vi "Acquisition_BassShaker.vi"() -> ()   [LabVIEW 2017]
uses:
  <vilib>/Utility/error.llb/DialogType.ctl
  <vilib>/DAQmx/write.llb/DAQmx Write (Digital Bool 1Line 1Point).vi
  <vilib>/DAQmx/read.llb/DAQmx Read (Analog 1D Wfm NChan NSamp).vi
  <vilib>/Utility/file.llb/Write Delimited Spreadsheet (DBL).vi
panel:
  in  "Activity Based On:":u16(ring) items=["EMG", "Piezo"]
  in  "Piezo Filter Parameters File:":path=path "C:/Users/local_admin/Desktop/Sleep Modulation/Piezo_Coefs.csv"
  in  "AO Channel":tag="Dev3/ao0"
  out "Stim":bool
  in  "Stim?":bool
  out "Detection":bool
  in  "Stop":bool
  in  "Target State:":u16(ring)=3 items=["Wake"=1, "NREM"=2, "REM"=3]
  in  "Frequency":dbl=50.0 format="%0.2p"
  in  "Amplitude":dbl=0.2 format="%0.2p"
  in  "Preamp Gain:":u16(ring)=10 items=["10X"=10, "100X"=100]
  in  "Modeling":u16(ring)=1 items=["Building", "Implementing"]
  out "Predicted State":i32(ring)=1 items=["Wake"=1, "NREM"=2, "REM"=3]
  in  "Minimum\nDuration":dbl=5.0
  in  "Feature Save To Path":path=path "C:/Users/local_admin/Desktop/Shaker Trials/NSL39/50Hz, 200mV/NSL39_50Hz200mV.csv"
  in  "EEG Filter Parameters File:":path=path "C:/Users/local_admin/Desktop/Sleep Modulation/EEG_Coefs.csv"
  in  "Model Information File (Mu, Sigma, Priors, Transition Matrix):":path=path "C:/Users/local_admin/Desktop/Shaker Trials/NSL39/Model_NSL39_10072017.csv"
  out "EEG":waveform(dbl)(graph)={"t0"=timestamp(3591178838.0438023 s since 1904-01-01), "dt"=0.0025, "Y"=array[400 elements], "attributes"=variant("NI_ChannelName"=variant(string "EEG"), "NI_UnitDescription"=variant(string "Volts"))}
  out "Piezo":waveform(dbl)(graph)={"t0"=timestamp(0 s since 1904-01-01), "dt"=1.0, "Y"=array[400 elements]}
  # "STIMULATION SETTINGS"
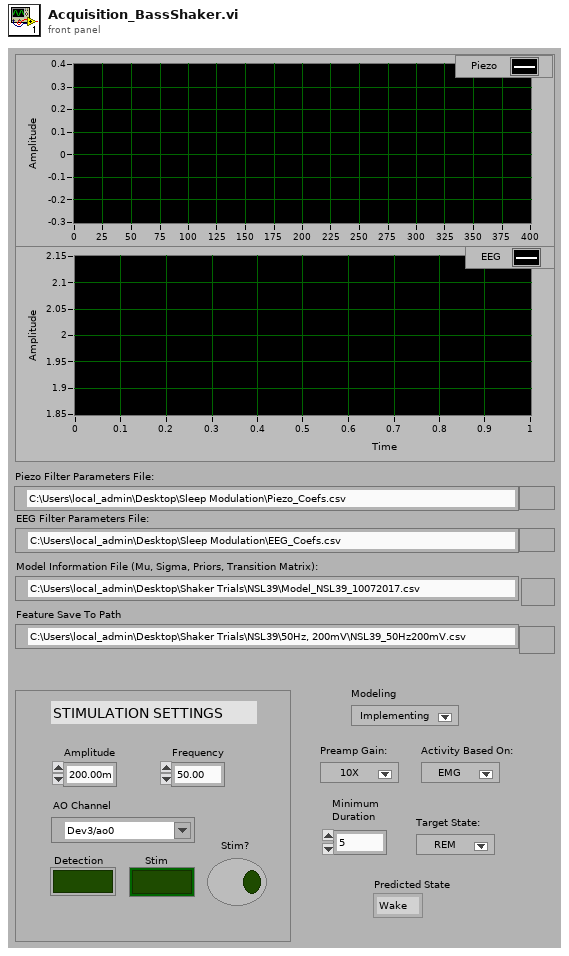
[diagram p1: front panel]
types:
  T1 = typedef "DialogType.ctl" = u16
  T2 = typedef "TYPE EEG Components.ctl" = cluster{"Total":dbl, "Alpha":dbl, "Beta":dbl, "Gamma":dbl, "Delta":dbl, "Delta Low":dbl, "Delta High":dbl, "Theta":dbl}
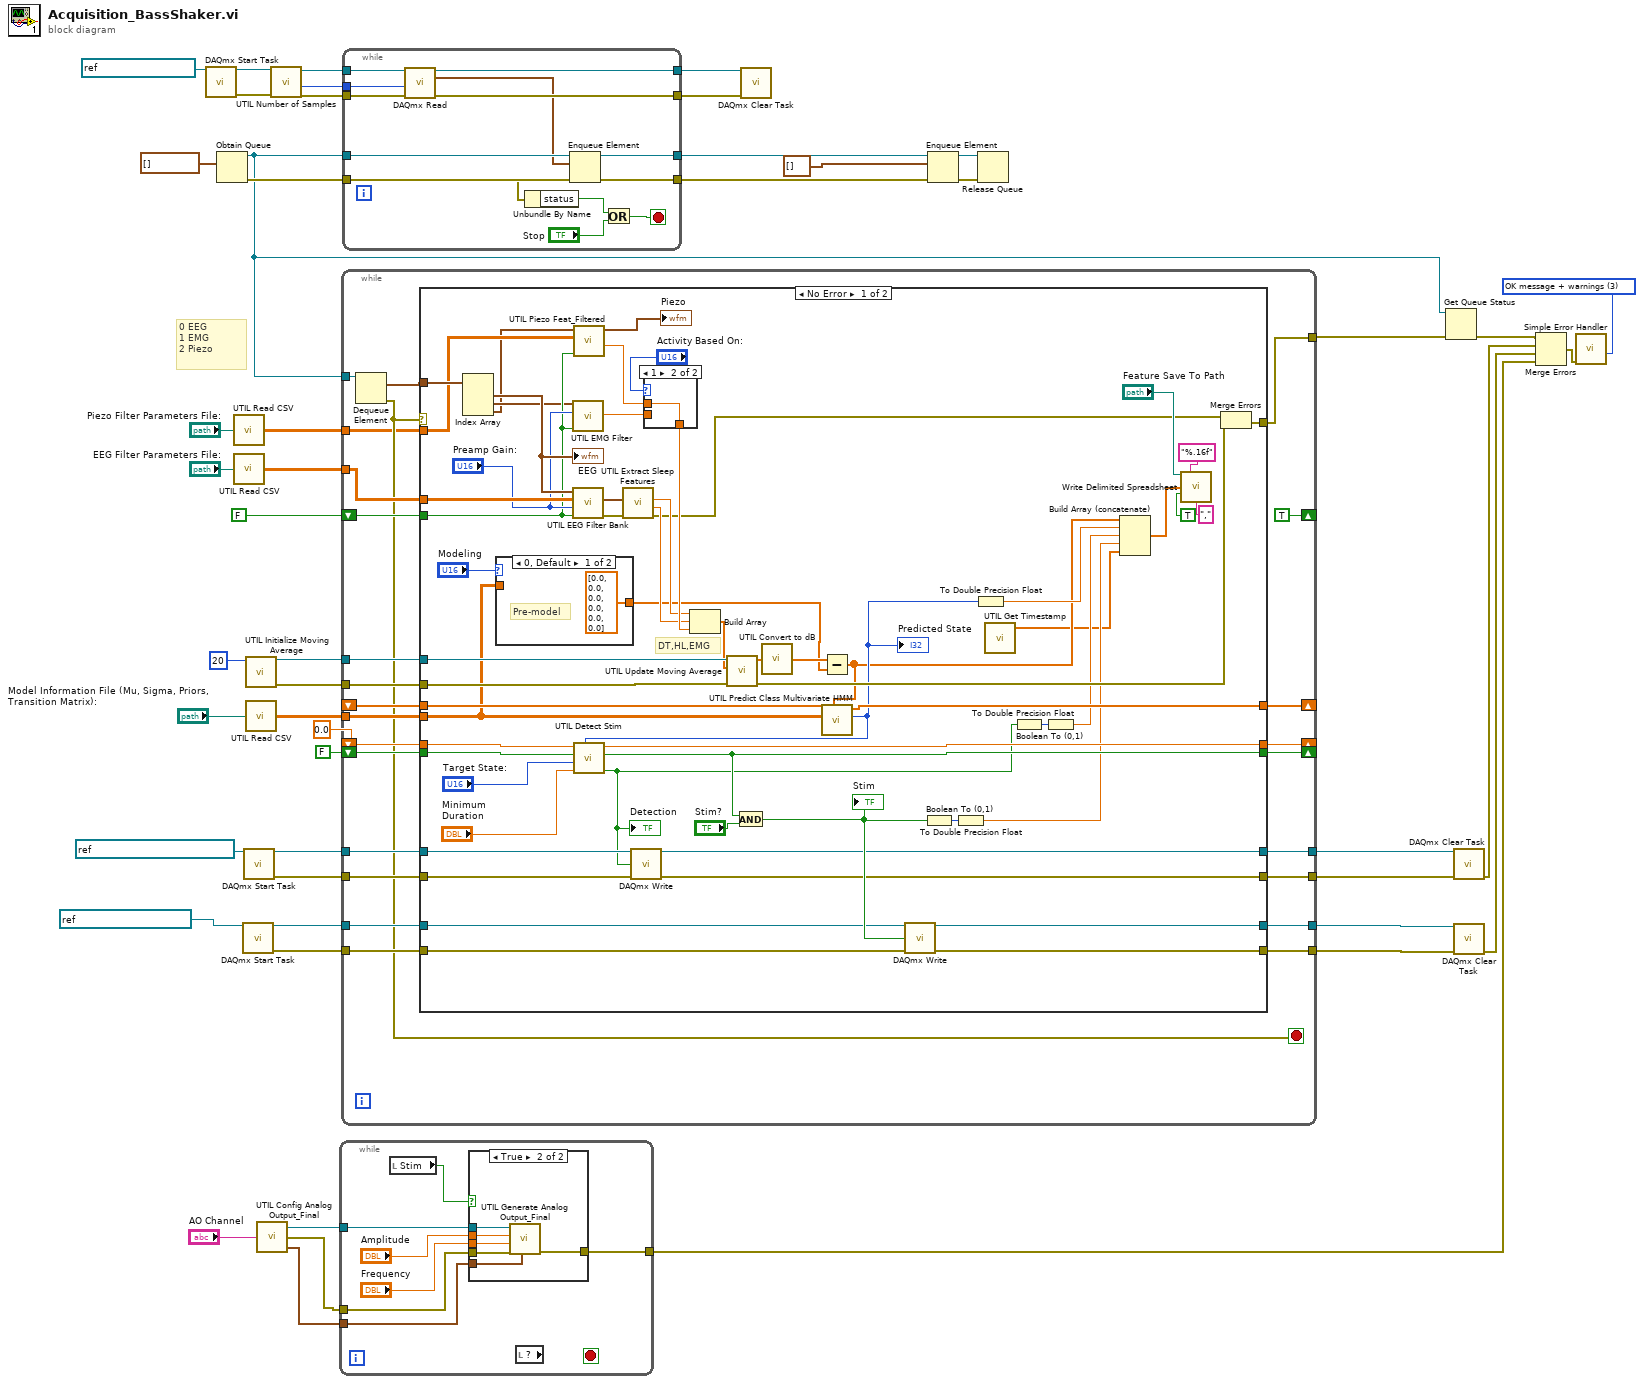
[diagram p0: block diagram]
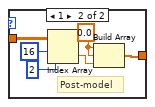
[diagram p3: hidden frame]
diagram:
  w42 = T1 3 items=["no dialog", "OK message", "continue or stop message", "OK message + warnings", "continue/stop + warnings"] ("type of dialog (OK msg:1)")
  # "0 EEG\n1 EMG\n2 Piezo"
  n1 = call <vilib>:"DAQmx Start Task.vi"("task/channels in"=refnum<k21> "BassShakerInput") -> ("task out"=w37:refnum<k21>, "error out"=w36:errorcluster)  [unwired: 13 in]
  n2 = Obtain Queue(element data type=waveform(dbl)[] [] ("Measurement 2")) -> (queue out=w3:refnum<queue>, error out=w48:errorcluster)  [unwired: 4 in, 1 out]
  n3 = call "UTIL Read CSV.vi"("CSV Path"="Piezo Filter Parameters File:") -> ("Data From File"=w1:dbl[][])
  n4 = call "UTIL Read CSV.vi"("CSV Path"="EEG Filter Parameters File:") -> ("Data From File"=w26:dbl[][])
  n5 = call <vilib>:"DAQmx Start Task.vi"("task/channels in"=refnum<k21> "StimAnnotationOut") -> ("task out"=w20:refnum<k21>, "error out"=w19:errorcluster)  [unwired: 13 in]
  n6 = call <vilib>:"DAQmx Start Task.vi"("task/channels in"=refnum<k21> "DetectionAnnotationOut") -> ("task out"=w23:refnum<k21>, "error out"=w22:errorcluster)  [unwired: 13 in]
  n7 = call "UTIL Initialize Moving Average.vi"("Window Width"=20) -> ("Error Out"=w29:errorcluster, "queue out"=w27:refnum<queue>)  [unwired: 9 in]
  n8 = call "UTIL Read CSV.vi"("CSV Path"="Model Information File (Mu, Sigma, Priors, Transition Matrix):") -> ("Data From File"=w39:dbl[][])
  n9 = call "UTIL Config Analog Output_Final.vi"("physical channels"="AO Channel") -> ("sampling info"=w10:cluster{"Fs":dbl, "#s":dbl}, "error out"=w8:errorcluster, "task out"=w7:refnum<k21>)
  n10 = call "UTIL Number of Samples.vi"("Error In"=w36, "Task In"=w37) -> ("Error Out"=w32:errorcluster, "Samples/Chan"=w33:i32, "Task Out"=w34:refnum<k21>)  [unwired: 7 in]
  n11 = while {
    tunnel: w10 -> [w54]
    tunnel: w8 -> [w53]
    tunnel: w7 -> [w52]
    tunnel: [w51] -> w6
    stop <- _ stop-if-true
    n12 = local read "Stim"() -> (w50:bool)
    n13 = case shown="True" w50 {
      tunnel: "Amplitude" -> [_ w63]
      tunnel: "Frequency" -> [_ w62]
      tunnel: w54 -> [_ w61]
      tunnel: w53 -> [w57 w60]
      tunnel: w52 -> [_ w59]
      tunnel: [w57 w58] -> w51
      frame False {
      }
      frame True {
        n14 = call "UTIL Generate Analog Output_Final.vi"("sampling info"=w61, "error in (no error)"=w60, "frequency"=w62, "amplitude"=w63, "task/channels in"=w59) -> ("error out"=w58:errorcluster)  [unwired: 5 in, 1 out]
      }
    }
    n15 = local read item#-1() -> ()  [unwired: 1 out]
  }
  n16 = while {
    tunnel: w3 -> [w87]
    shift-right: [TRUE] -> _
    shift-left: FALSE -> [w85]
    tunnel: [w81] -> w4
    tunnel: w29 -> [w84]
    tunnel: w39 -> [w83]
    tunnel: w26 -> [w82]
    tunnel: w27 -> [w80]
    shift-right: [w79] -> _
    shift-left: _ -> [w78]
    shift-right: [w76] -> _
    shift-left: 0.0 ("Detection Duration Out") -> [w77]
    shift-right: [w74] -> _
    shift-left: FALSE ("Stim State Out") -> [w75]
    tunnel: w23 -> [w73]
    tunnel: w22 -> [w72]
    tunnel: w20 -> [w71]
    tunnel: w19 -> [w70]
    tunnel: [w69] -> w18
    tunnel: [w68] -> w17
    tunnel: [w67] -> w16
    tunnel: [w66] -> w15
    tunnel: w1 -> [w64]
    stop <- w65 stop-if-true
    n17 = Dequeue Element(queue=w87) -> (element=w88:waveform(dbl)[], error out=w65:errorcluster)  [unwired: 2 in, 2 out]
    n18 = case shown="No Error" w65 {
      selector: w65 -> [_ w158]
      tunnel: w88 -> [w128 _]
      tunnel: w85 -> [w94 _]
      tunnel: [w142 w158] -> w81
      tunnel: w84 -> [w139 _]
      tunnel: w83 -> [w127 _]
      tunnel: w82 -> [w141 _]
      tunnel: w80 -> [w137 _]
      tunnel: [w136 w165] -> w79
      tunnel: w78 -> [w135 w165]
      tunnel: w77 -> [w123 w160]
      tunnel: [w122 w160] -> w76
      tunnel: w75 -> [w121 w159]
      tunnel: [w108 w159] -> w74
      tunnel: w73 -> [w119 w162]
      tunnel: w72 -> [w118 w161]
      tunnel: w71 -> [w114 w164]
      tunnel: w70 -> [w113 w163]
      tunnel: [w112 w164] -> w69
      tunnel: [w111 w163] -> w68
      tunnel: [w110 w162] -> w67
      tunnel: [w109 w161] -> w66
      tunnel: w64 -> [w95 _]
      frame No Error {
        # "DT,HL,EMG"
        n19 = Index Array(array=w128) -> (element #1=w106:waveform(dbl), element #2=w91:waveform(dbl), element #3=w90:waveform(dbl))  [unwired: 3 in]
        "EEG" <- w106
        n20 = case shown="0, Default" "Modeling" {
          tunnel: w127 -> [_ w155]
          tunnel: [dbl[] [0.0, 0.0, 0.0, 0.0, 0.0, 0.0] ("Parameters Out") w154] -> w125
          frame 0, Default {
            # "Pre-model"
          }
          frame 1 {
            w150 = 0.0 ("element")
            # "Post-model"
            n21 = Index Array(array=w155, index (row)=16, index (col)=2 ("disabled index (col)")) -> (element=w151:dbl)
            n22 = Build Array(w150, w150, w151) -> (w154:dbl[])
          }
        }
        n23 = call "UTIL EMG Filter.vi"("init/cont (init:F)"=w94, "Preamp Gain"="Preamp Gain:", "EMG In"=w91) -> ("EMG Power"=w134:dbl)  [unwired: 7 in, 1 out]
        n24 = call "UTIL EEG Filter Bank.vi"("init/cont (init:F)"=w94, "Amplifier Gain"="Preamp Gain:", "Filter Coefficients from File"=w141, "EEG In"=w106) -> ("Error Out"=w148:errorcluster, "EEG Components"=w140:T2)  [unwired: 5 in, 1 out]
        n25 = call "UTIL Piezo Feat_Filtered.vi"("Init/Cont?"=w94, "Filter Coefficients from File"=w95, "Piezo In"=w90) -> ("Piezo Power"=w96:dbl, "Filtered Piezo Out"=→"Piezo":waveform(dbl))  [unwired: 3 in]
        n26 = call "UTIL Extract Sleep Features.vi"("Error In"=w148, "Components In"=w140) -> ("Error Out"=w105:errorcluster, "Hi:Lo"=w132:dbl, "Delta:Theta"=w131:dbl)  [unwired: 6 in, 1 out]
        n27 = case shown="1" "Activity Based On:" {
          tunnel: w134 -> [w156 _]
          tunnel: w96 -> [_ w157]
          tunnel: [w156 w157] -> w133
          frame 0, Default {
          }
          frame 1 {
          }
        }
        n28 = Build Array(w131, w132, w133) -> (w130:dbl[])
        n29 = call "UTIL Update Moving Average.vi"("Error In"=w139, "Data In"=w130, "Average Queue"=w137) -> ("Error Out"=w138:errorcluster, "Average"=w129:dbl[])  [unwired: 7 in]
        n30 = call "UTIL Convert to dB.vi"("Features In"=w129) -> ("Features (dB)"=w126:dbl[])
        n31 = Subtract(x=w126, y=w125) -> (x-y=w103:dbl[])
        n32 = call "UTIL Predict Class Multivariate HMM.vi"("Data Point"=w103, "Model Information"=w127, "d(t-1) In"=w135) -> ("Sleep Stage"=w107:i32, "d(t-1) Out"=w136:dbl[])  [unwired: 5 in]
        "Predicted State" <- w107
        n33 = call "UTIL Detect Stim.vi"("Predicted State"=w107, "Min Duration"="Minimum\nDuration", "Target State"="Target State:", "Previous Stim State"=w121, "Detection Duration In"=w123) -> ("Detection"=w92:bool, "Stim State Out"=w108:bool, "Detection Duration Out"=w122:dbl)  [unwired: 4 in]
        "Detection" <- w92
        n34 = call-poly <vilib>:"DAQmx Write.vi"("task/channels in"=w119, "data"=w92, "error in"=w118) -> ("task out"=w110:refnum<k21>, "error out"=w109:errorcluster)  [unwired: 10 in, 1 out]
        n35 = And(x=w108, y="Stim?") -> (x .and. y?=w115:bool)
        "Stim" <- w115
        n36 = call-poly <vilib>:"DAQmx Write.vi"("task/channels in"=w114, "data"=w115, "error in"=w113) -> ("task out"=w112:refnum<k21>, "error out"=w111:errorcluster)  [unwired: 10 in, 1 out]
        n37 = Boolean To (0,1)(Boolean=w115) -> (0, 1=w116:i16)
        n38 = To Double Precision Float(number=w116) -> (double precision float=w101:dbl)
        n39 = To Double Precision Float(number=w107) -> (double precision float=w143:dbl)
        n40 = call "UTIL Get Timestamp.vi"() -> ("appended array"=w100:dbl[])  [unwired: 7 in, 1 out]
        n41 = Boolean To (0,1)(Boolean=w92) -> (0, 1=w120:i16)
        n42 = To Double Precision Float(number=w120) -> (double precision float=w102:dbl)
        n43 = Build Array (concatenate)(w103, w143, w102, w101, w100) -> (w144:dbl[])
        n44 = call-poly <vilib>:"Write Delimited Spreadsheet.vi"("file path (dialog if empty)"="Feature Save To Path", "format (%.3f)"="%.16f", "1D data"=w144, "append to file? (new file:F)"=TRUE, "delimiter (\\t)"="," ("delimiter (\\t)")) -> ()  [unwired: 9 in, 2 out]
        n45 = Merge Errors(w105, w138) -> (w142:errorcluster)
      }
      frame Error {
      }
    }
  }
  n46 = while {
    tunnel: [w178] -> w31
    tunnel: w3 -> [w177]
    tunnel: w48 -> [w176]
    tunnel: [w170] -> w46
    tunnel: [w169] -> w45
    tunnel: w34 -> [w175]
    tunnel: w33 -> [w174]
    tunnel: w32 -> [w173]
    tunnel: [w172] -> w30
    stop <- w166 stop-if-true
    n47 = call-poly <vilib>:"DAQmx Read.vi"("task/channels in"=w175, "number of samples per channel"=w174, "error in"=w173) -> ("task out"=w178:refnum<k21>, "data"=w171:waveform(dbl)[], "error out"=w172:errorcluster)  [unwired: 10 in]
    n48 = Enqueue Element(queue=w177, element=w171, error in (no error)=w176) -> (queue out=w170:refnum<queue>, error out=w169:errorcluster)  [unwired: 1 in, 1 out]
    n49 = Unbundle By Name(w169) -> ("status"=w167:bool)
    n50 = Or(x=w167, y="Stop") -> (x .or. y?=w166:bool)
  }
  n51 = call <vilib>:"DAQmx Clear Task.vi"("task in"=w31, "error in"=w30) -> ()  [unwired: 13 in, 1 out]
  n52 = Enqueue Element(queue=w46, element=waveform(dbl)[] [] ("Measurement 2"), error in (no error)=w45) -> (queue out=w43:refnum<queue>, error out=w41:errorcluster)  [unwired: 1 in, 1 out]
  n53 = Release Queue(queue=w43, error in (no error)=w41) -> ()  [unwired: 1 in, 3 out]
  n54 = Get Queue Status(queue=w3, error in (no error)=w4) -> (error out=w5:errorcluster)  [unwired: 1 in, 7 out]
  n55 = call <vilib>:"DAQmx Clear Task.vi"("task in"=w16, "error in"=w15) -> ("error out"=w14:errorcluster)  [unwired: 13 in]
  n56 = call <vilib>:"DAQmx Clear Task.vi"("task in"=w18, "error in"=w17) -> ("error out"=w13:errorcluster)  [unwired: 13 in]
  n57 = Merge Errors(w5, w14, w13, w6) -> (w38:errorcluster)
  n58 = call <vilib>:"Simple Error Handler.vi"("type of dialog (OK msg:1)"=w42, "error in (no error)"=w38) -> ()  [unwired: 3 in, 5 out]
